vi "genNewFilePathFromCounter.vi"(8 "error in (no error)":errorcluster, 10 "filePathOld":path, 11 "Logger in":refnum<class "Logger.lvclass">) -> (0 "error out":errorcluster, 2 "filePathNew":path, 3 "Logger out":refnum<class "Logger.lvclass">)   [LabVIEW 2018, in "Logger.lvclass"]
doc: "Generate the new file path from the counter of file. The counter of file will be added by 1."
uses:
  Logger.lvclass
  Logger.lvclass/Logger.ctl
  <vilib>/regexp/Match Regular Expression.xnode
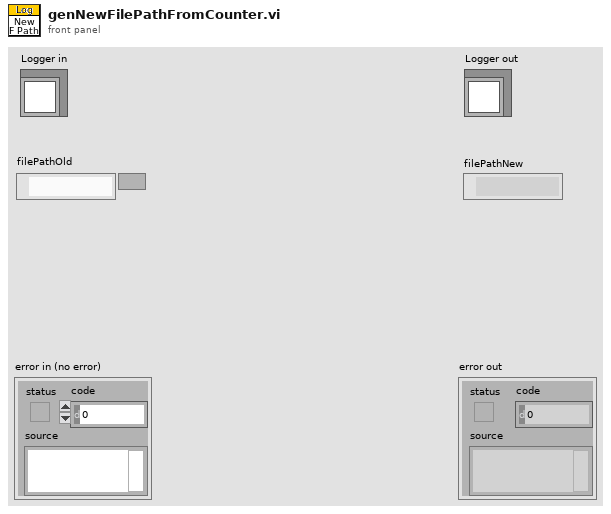
[diagram p1: front panel]
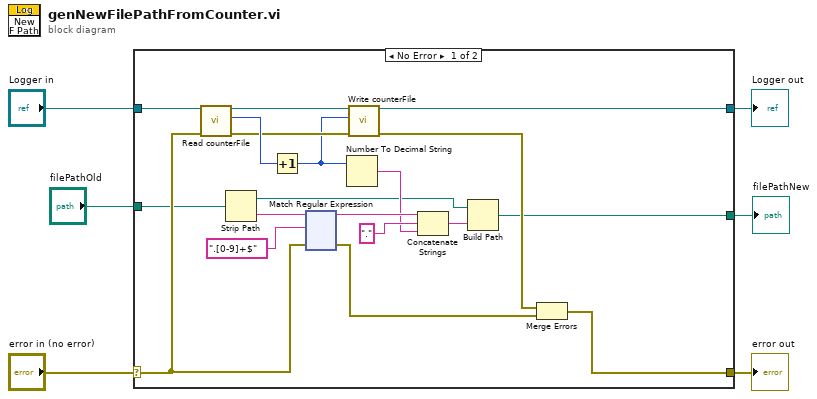
[diagram p0: block diagram]
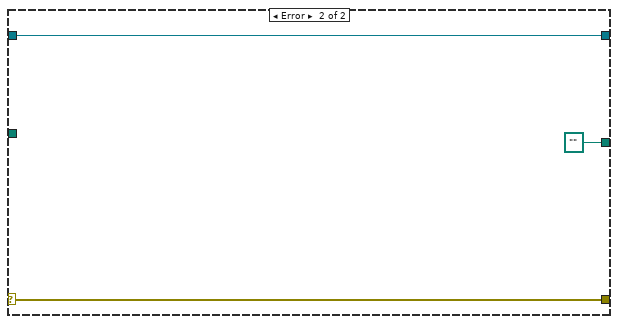
[diagram p2: hidden frame]
diagram:
  n1 = case shown="No Error" "error in (no error)" {
    selector: "error in (no error)" -> [w10 w142]
    tunnel: [w9 w142] -> w5
    tunnel: [w11 w141] -> w3
    tunnel: "Logger in" -> [w12 w141]
    tunnel: [w8 path "" ("appended path")] -> w2
    tunnel: "filePathOld" -> [w7 _]
    frame No Error {
      n2 = call "Read counterFile.vi"("error in (no error)"=w10, "Logger in"=w12) -> ("error out"=w22:errorcluster, "counterFile"=w24:u32, "Logger out"=w23:refnum<class "Logger.lvclass">)  [unwired: 7 in]
      n3 = Strip Path(path=w7) -> (stripped path=w15:path, name=w25:string)
      n4 = Increment(x=w24) -> (x+1=w18:u32)
      n5 = xnode "Match Regular Expression"("input string"=w25, "regular expression"=".[0-9]+$", "error in"=w10) -> ("before match"=w20:string, "error out"=w13:errorcluster)  [unwired: 3 in, 3 out]
      n6 = Number To Decimal String(number=w18) -> (decimal integer string=w17:string)  [unwired: 1 in]
      n7 = call "Write counterFile.vi"("error in (no error)"=w22, "counterFile"=w18, "Logger in"=w23) -> ("error out"=w14:errorcluster, "Logger out"=w11:refnum<class "Logger.lvclass">)  [unwired: 7 in]
      n8 = Concatenate Strings(w20, "." ("string"), w17) -> (w16:string)
      n9 = Build Path(base path=w15, name or relative path=w16) -> (appended path=w8:path)
      n10 = Merge Errors(w14, w13) -> (w9:errorcluster)
    }
    frame Error {
    }
  }
  "error out" <- w5
  "Logger out" <- w3
  "filePathNew" <- w2
